vi "Convert to JSON Comp Format.vi"(11 "digital audio protocol settings":T2) -> (3 "JSON compatible settings":T1)   [LabVIEW 2021, in "digital audio protocol controls.lvlib"]
uses:
  digital audio protocol controls.lvlib
  digital audio protocol settings.ctl
  digital audio protocol settings_json.ctl
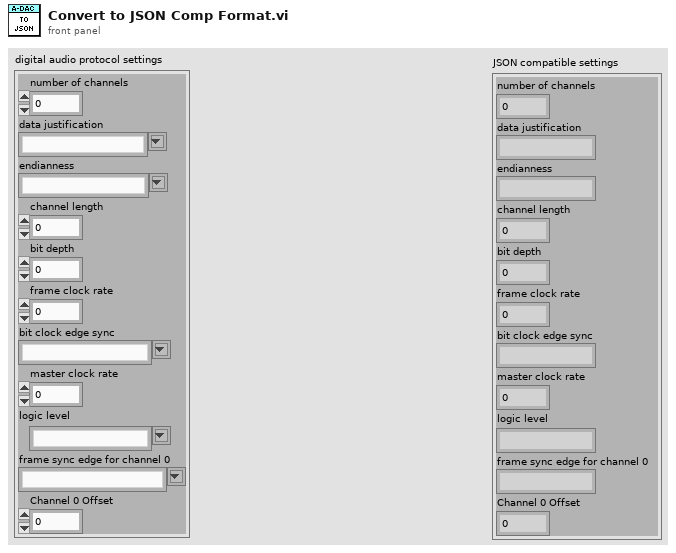
[diagram p1: front panel]
types:
  T1 = typedef "digital audio protocol controls.lvlib/digital audio protocol settings_json.ctl" = cluster{"number of channels":u32, "data justification":string, "endianness":string, "channel length":u32, "bit depth":u32, "frame clock rate":dbl, "bit clock edge sync":string, "master clock rate":dbl, "logic level":string, "frame sync edge for channel 0":string, "Channel 0 Offset":u32}
  T2 = typedef "digital audio protocol controls.lvlib/digital audio protocol settings.ctl" = cluster{"number of channels":u32, "data justification":string, "endianness":string, "channel length":u32, "bit depth":u32, "frame clock rate":dbl, "bit clock edge sync":string, "master clock rate":dbl, "logic level":string, "frame sync edge for channel 0":string, "Channel 0 Offset":u32}
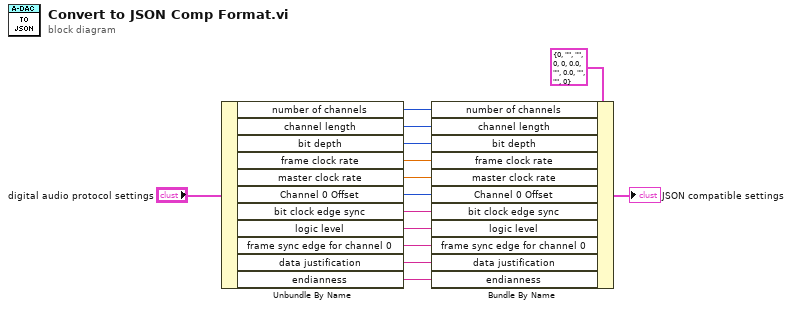
[diagram p0: block diagram]
diagram:
  n1 = Unbundle By Name("digital audio protocol settings") -> ("number of channels"=w11:u32, "channel length"=w10:u32, "bit depth"=w9:u32, "frame clock rate"=w8:dbl, "master clock rate"=w7:dbl, "Channel 0 Offset"=w6:u32, "bit clock edge sync"=w5:string, "logic level"=w4:string, "frame sync edge for channel 0"=w3:string, "data justification"=w2:string, "endianness"=w1:string)
  n2 = Bundle By Name(cluster=T1 {"number of channels"=0, "data justification"="", "endianness"="", "channel length"=0, "bit depth"=0, "frame clock rate"=0.0, "bit clock edge sync"="", "master clock rate"=0.0, "logic level"="", "frame sync edge for channel 0"="", "Channel 0 Offset"=0} ("JSON compatible settings"), "number of channels"=w11, "channel length"=w10, "bit depth"=w9, "frame clock rate"=w8, "master clock rate"=w7, "Channel 0 Offset"=w6, "bit clock edge sync"=w5, "logic level"=w4, "frame sync edge for channel 0"=w3, "data justification"=w2, "endianness"=w1) -> (→"JSON compatible settings":T1)
